vi "Shifter control.vi"(1 "High":bool, 2 "Low":bool) -> ()   [LabVIEW 2013]
uses:
  Events.vi
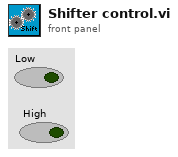
[diagram p1: front panel]
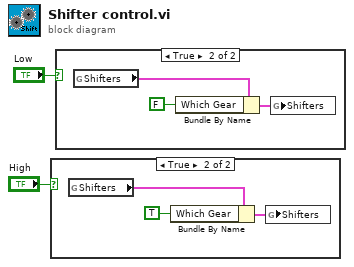
[diagram p0: block diagram]
diagram:
  n1 = case shown="True" "High" {
    frame False {
    }
    frame True {
      n2 = global read "Events.vi" "Shifters"() -> (w4:cluster{"Which Gear":bool})
      n3 = Bundle By Name(cluster=w4, "Which Gear"=TRUE) -> (w5:cluster{"Which Gear":bool})
      n4 = global write "Events.vi" "Shifters"(w5) -> ()
    }
  }
  n5 = case shown="True" "Low" {
    frame False {
    }
    frame True {
      n6 = global read "Events.vi" "Shifters"() -> (w7:cluster{"Which Gear":bool})
      n7 = Bundle By Name(cluster=w7, "Which Gear"=FALSE) -> (w8:cluster{"Which Gear":bool})
      n8 = global write "Events.vi" "Shifters"(w8) -> ()
    }
  }
